vi "Bertta_v06.vi"() -> ()   [LabVIEW 2015]
uses:
  BERTTA.dll
panel:
  out "Mettler 3":dbl(graph)
  out "Mettler 2":dbl(graph)
  in  "PAUSE":bool
  in  "?":bool
  in  "Tab Control":T1(tab)
  in  "Description":string
  in  "Project name":string
  in  "User (initials)":string
  out "Mettler 1":dbl(graph)
  out "?":dbl(graph)
  in  "Balances":bool[](array[boolean])
  out "Waveform Chart 3":dynamicdata(graph)
  out "Table":string[][](table)
  in  "Headers":string[](array[string])
  in  "?":bool
  in  "Seq":dbl[][](array[numeric])=[[20.0, 60.0, 40.0], [60.0, 40.0, 20.0], [100.0, 100.0, 100.0]]
  out "Elapsed":i32
  out "Step":i32
  out "Sp":dbl
  out "T":dbl
  out "Tinit":dbl
  out "Tset":dbl
  out "Time constant":dbl
  out "Sp - Tset":i32
  out "Change":i32
  out "Waveform Chart":dynamicdata(graph)
  in  "Tbypass":dbl=33.0
  in  "Tfail":dbl=22.0
  in  "err":i32
  out "Waveform Chart 2":dynamicdata(graph)
  out "Rate (g/s)":dbl
  out "Time (s)":dbl
  out "Target (g)":dbl
  in  "Seq 2":dbl[][](array[numeric])=[[20.0, 60.0, 40.0], [60.0, 40.0, 20.0], [100.0, 100.0, 100.0]]
  out "Weight (1)":dbl
  out "target reached":i32
  out "x/y":dbl
  out "bal_previous":i32
  out "Step":i32
  in  "?":bool
  out "Step":i32
  out "bal_previous":i32
  out "x/y":dbl
  out "target reached":i32
  out "Waveform Chart 5":dynamicdata(graph)
  out "Weight (2)":dbl
  out "Rate (g/s)":dbl
  out "Time (s)":dbl
  out "Target (g)":dbl
  in  "Seq 3":dbl[][](array[numeric])=[[20.0, 60.0, 40.0], [60.0, 40.0, 20.0], [100.0, 100.0, 100.0]]
  in  "Boolean":bool
  out "Step":i32
  out "bal_previous":i32
  out "x/y":dbl
  out "target reached":i32
  out "Waveform Chart 6":dynamicdata(graph)
  out "Weight (3)":dbl
  out "Rate (g/s)":dbl
  out "Time (s)":dbl
  out "Target (g)":dbl
  in  "Seq 4":dbl[][](array[numeric])=[[20.0, 60.0, 40.0], [60.0, 40.0, 20.0], [100.0, 100.0, 100.0]]
  out "RPM":dbl
  out "Waveform Chart 4":dynamicdata(graph)
  in  "Set RPM":dbl(slide) scale=0.0..500.0
  out "Torque":dbl
  in  "?":T2(tab)
  in  "Device port":dbl=1.0
  out "Debug msg":dbl
  in  "Device port":dbl=20.0
  in  "Device port":i32=2
  in  "Device port 2":i32=6
  in  "Device port 3":i32=6
  in  "Device port 4":i32=1
  # "1"
  # "2"
  # "3"
  # "4"
  # "Step 1"
  # "Step 2"
  # "Step 3"
  # "Step 4"
  # "Step 1"
  # "Step 2"
  # "Step 3"
  # "Step 4"
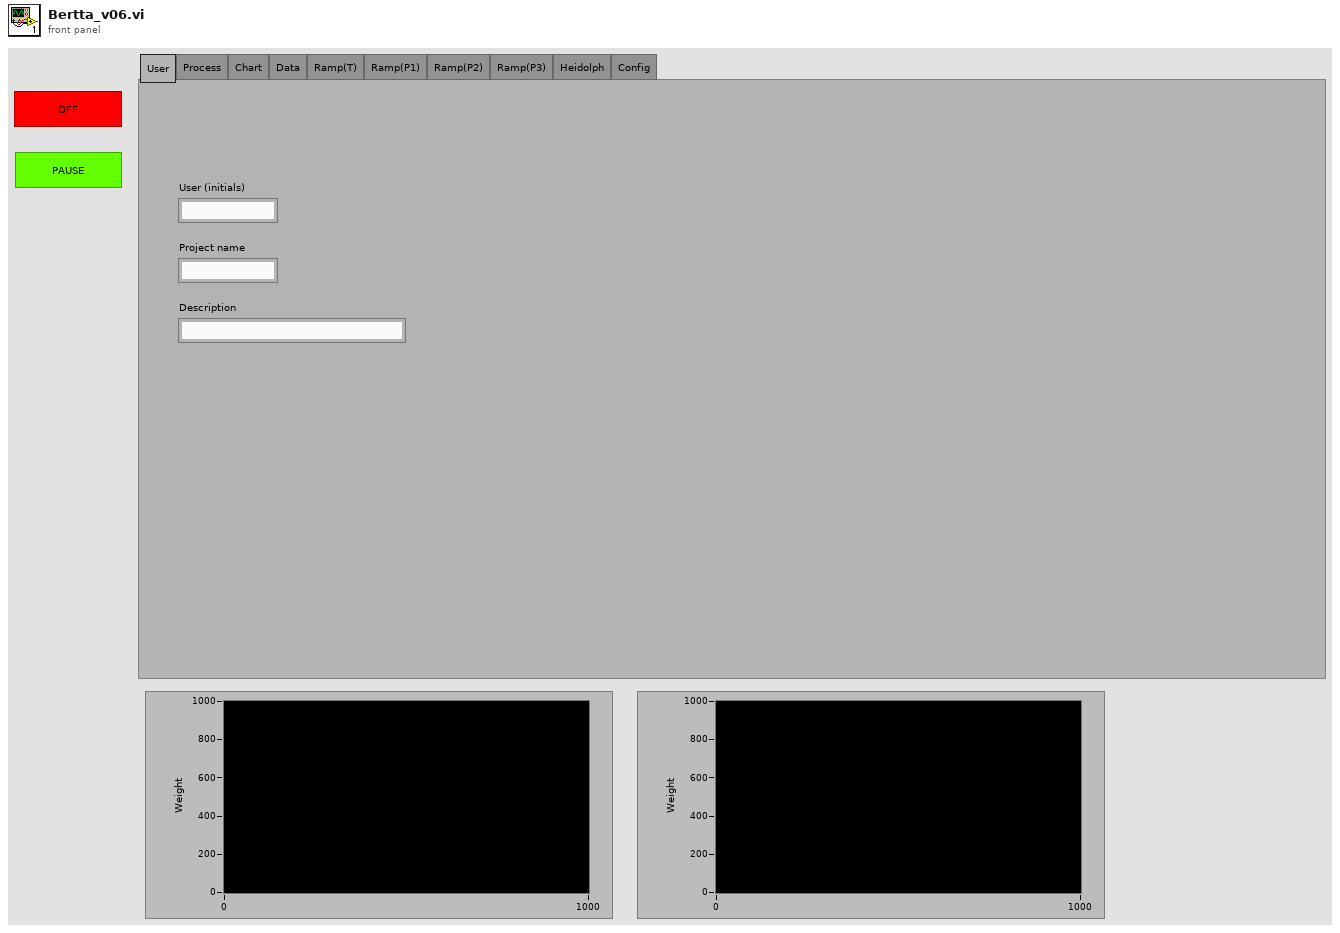
[diagram p1: front panel]
types:
  T1 = enum32{"User", "Process", "Chart", "Data", "Ramp(T)", "Ramp(P1)", "Ramp(P2)", "Ramp(P3)", "Heidolph", "Config"}
  T2 = enum32{"DB / File", "Lauda", "Heidolph", "Mettler 1", "Mettler 2", "Mettler 3", "Ismatec 1"}
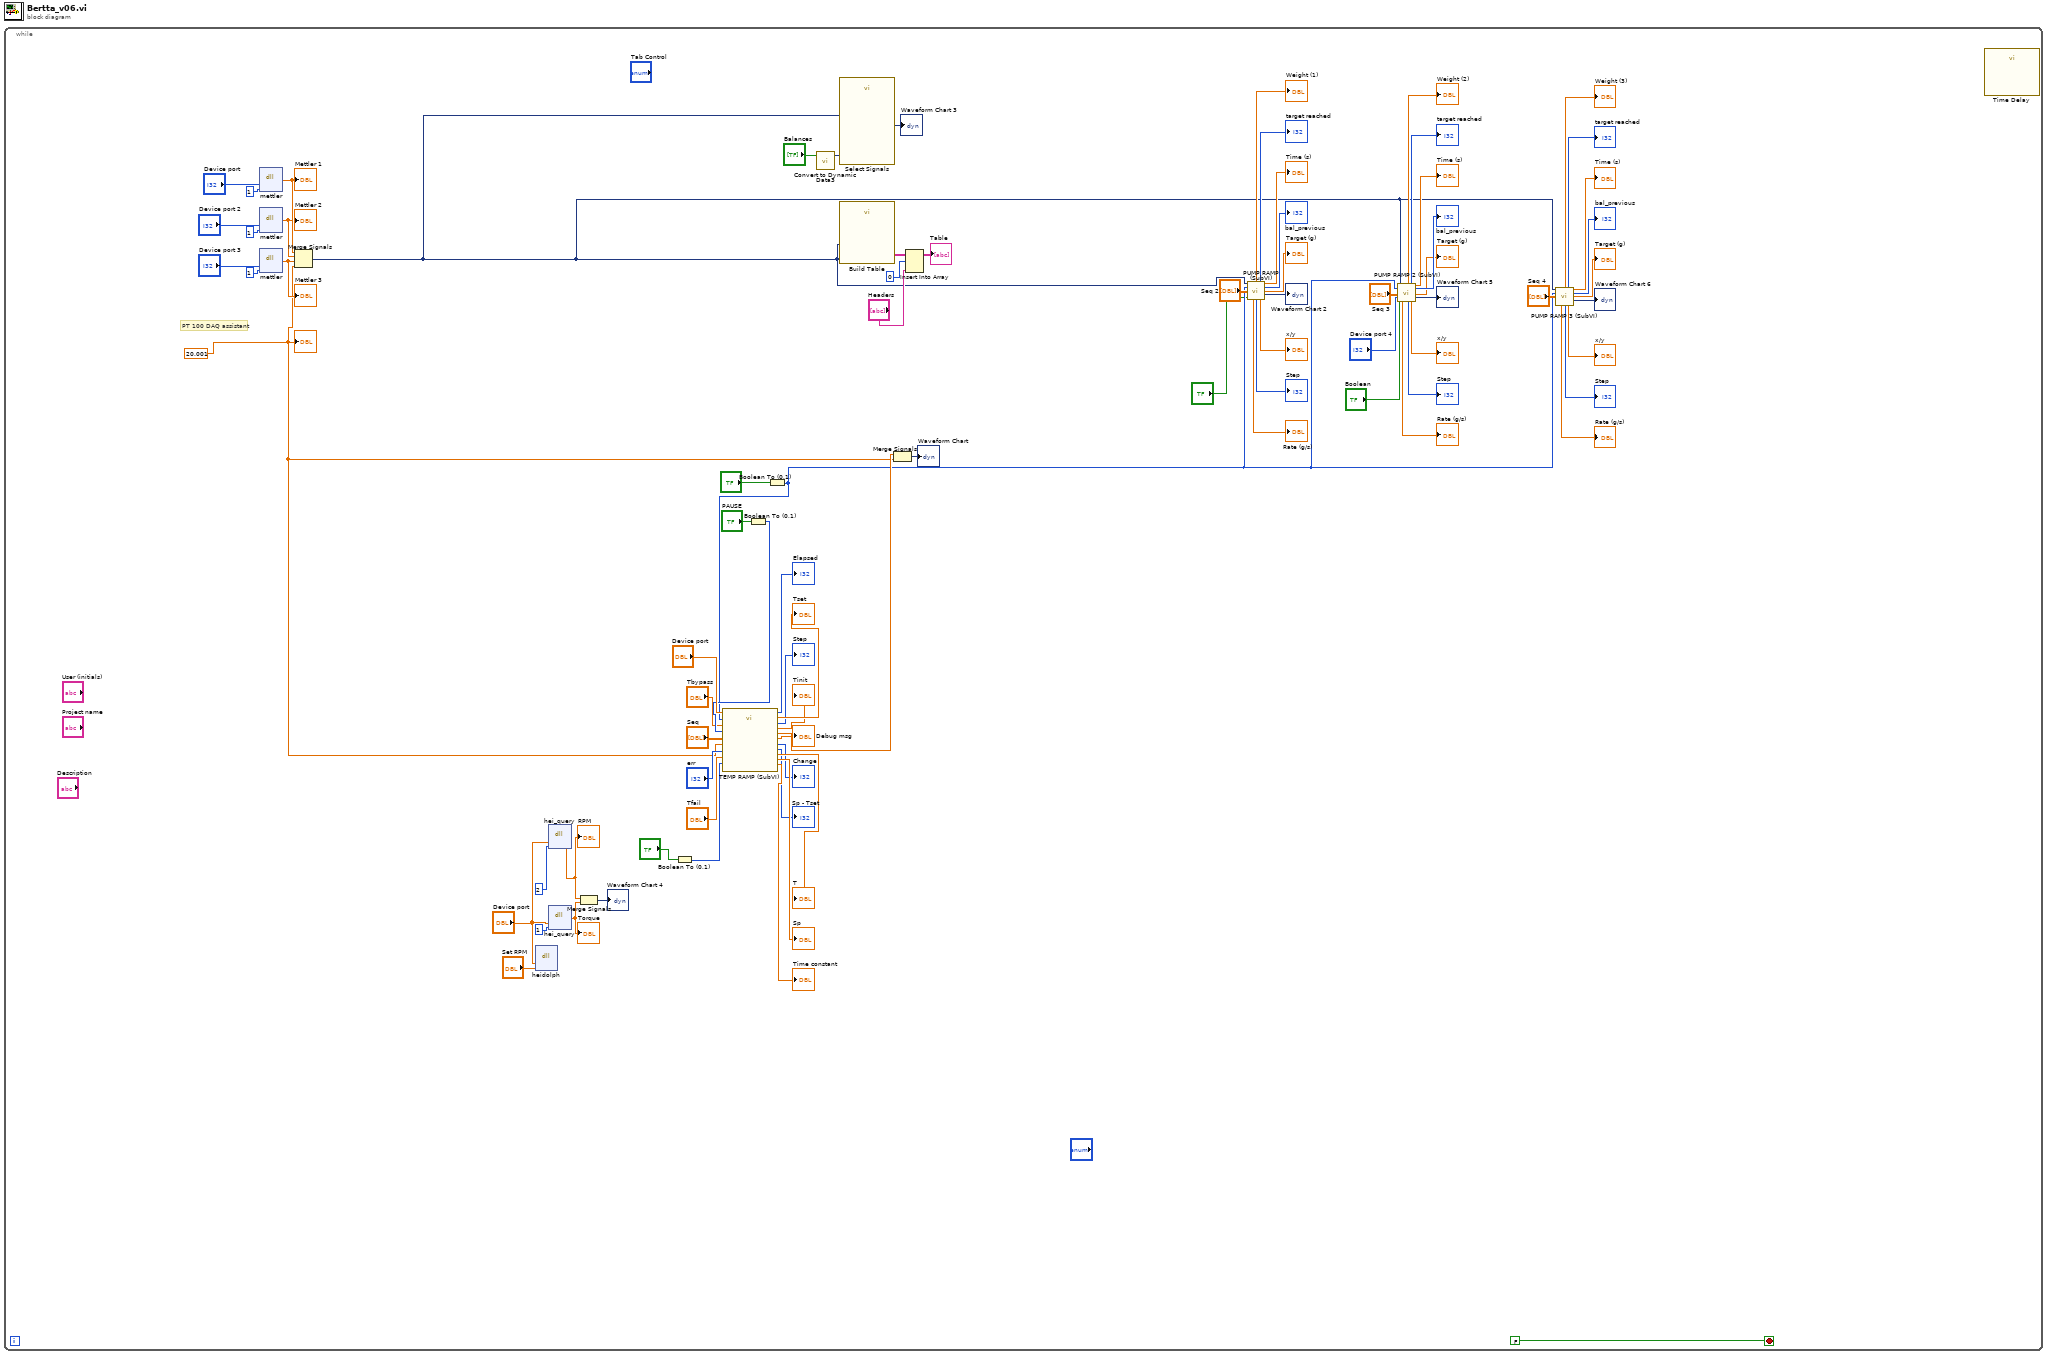
[diagram p0: block diagram]
diagram:
  n1 = while {
    stop <- FALSE stop-if-true
    w4 = 20.001
    # "PT 100 DAQ assistant"
    n2 = dll-call lib="C:/Users/xlaraser/Documents/Visual Studio 2017/Projects/Bertta/BERTTA/Debug/BERTTA.dll" fn="mettler"("port"="Device port", "msg"=1) -> ("return type"=w26:dbl)  [unwired: 5 in, 2 out]
    "Mettler 1" <- w26
    n3 = dll-call lib="C:/Users/xlaraser/Documents/Visual Studio 2017/Projects/Bertta/BERTTA/Debug/BERTTA.dll" fn="mettler"("port"="Device port 2", "msg"=1) -> ("return type"=w25:dbl)  [unwired: 5 in, 2 out]
    "Mettler 2" <- w25
    n4 = dll-call lib="C:/Users/xlaraser/Documents/Visual Studio 2017/Projects/Bertta/BERTTA/Debug/BERTTA.dll" fn="mettler"("port"="Device port 3", "msg"=1) -> ("return type"=w12:dbl)  [unwired: 5 in, 2 out]
    "Mettler 3" <- w12
    n5 = Merge Signals(w26, w25, w12, w4) -> (w5:dynamicdata)
    n6 = dll-call lib="C:/Users/xlaraser/Documents/Visual Studio 2017/Projects/Bertta/BERTTA/Debug/BERTTA.dll" fn="heidolph"("port"="Device port", "speed"="Set RPM") -> ()  [unwired: 6 in, 2 out]
    n7 = dll-call lib="C:/Users/xlaraser/Documents/Visual Studio 2017/Projects/Bertta/BERTTA/Debug/BERTTA.dll" fn="hei_query"("port"="Device port", "q"=2) -> ("return type"=w62:dbl)  [unwired: 5 in, 2 out]
    "RPM" <- w62
    n8 = dll-call lib="C:/Users/xlaraser/Documents/Visual Studio 2017/Projects/Bertta/BERTTA/Debug/BERTTA.dll" fn="hei_query"("port"="Device port", "q"=1) -> ("return type"=w61:dbl)  [unwired: 5 in, 2 out]
    "Torque" <- w61
    n9 = Merge Signals(w62, w61) -> (→"Waveform Chart 4":dynamicdata)
    n10 = Boolean To (0,1)(Boolean="?") -> (0, 1=w7:i16)
    n11 = Boolean To (0,1)(Boolean="PAUSE") -> (0, 1=w39:i16)
    n12 = Boolean To (0,1)(Boolean="?") -> (0, 1=w3:i16)
    n13 = call "TEMP RAMP (SubVI).vi"("Device port"="Device port", "Numeric"=w3, "Tbyp"="Tbypass", "Numeric 2"=w39, "Seq"="Seq", "data"=w4, "bypass"=w7, "err"="err", "Tfail"="Tfail") -> ("Sp - Tset"=→"Sp - Tset":i32, "T"=→"T":dbl, "Sp"=→"Sp":dbl, "Change"=→"Change":i32, "tr"=→"Time constant":dbl, "Debug msg"=→"Debug msg":dbl, "Elapsed"=→"Elapsed":i32, "Tset"=→"Tset":dbl, "Step"=→"Step":i32, "Tinit"=→"Tinit":dbl, "return type"=w68:dbl)
    n14 = call "Convert to Dynamic Data3"("Array"="Balances") -> ("Dynamic Data Type"=w73:dynamicdata)  [unwired: 3 in]
    n15 = call "Select Signals"("Selector Input"=w73, "Signals"=w5) -> ("Signal Out"=→"Waveform Chart 3":dynamicdata)  [unwired: 8 in, 1 out]
    n16 = call "Build Table"("Signals"=w5) -> ("Table"=w76:string[][])  [unwired: 4 in, 6 out]
    n17 = Merge Signals(w68, w4) -> (→"Waveform Chart":dynamicdata)
    n18 = Insert Into Array(array=w76, index (row)=0, new element="Headers") -> (→"Table":string[][])  [unwired: 1 in]
    n19 = call "PUMP RAMP (SubVI).vi"("Dynamic Data"=w5, "Numeric"=w3, "Seq in"="Seq 2", 11:"?") -> ("Weight (S1)"=→"Weight (1)":dbl, "target reached"=→"target reached":i32, "Time (s)"=→"Time (s)":dbl, "bal_previous"=→"bal_previous":i32, "Target (g)"=→"Target (g)":dbl, "Waveform Chart 2"=→"Waveform Chart 2":dynamicdata, "Rate (g/s)"=→"Rate (g/s)":dbl, "Step 2"=→"Step":i32, "x/y"=→"x/y":dbl)  [unwired: 3 in]
    n20 = call "PUMP RAMP 2 (SubVI).vi"("Dynamic Data"=w5, "Numeric"=w3, "Seq in"="Seq 3", "Device port"="Device port 4", "Boolean"="Boolean") -> ("Rate (g/s)"=→"Rate (g/s)":dbl, "Weight (S1)"=→"Weight (2)":dbl, "Step 2"=→"Step":i32, "target reached"=→"target reached":i32, "x/y"=→"x/y":dbl, "Time (s)"=→"Time (s)":dbl, "bal_previous"=→"bal_previous":i32, "Target (g)"=→"Target (g)":dbl, "Waveform Chart 2"=→"Waveform Chart 5":dynamicdata)  [unwired: 6 in]
    n21 = call "PUMP RAMP 3 (SubVI).vi"("Dynamic Data"=w5, "Numeric"=w3, "Seq in"="Seq 4") -> ("Weight (S1)"=→"Weight (3)":dbl, "target reached"=→"target reached":i32, "Time (s)"=→"Time (s)":dbl, "bal_previous"=→"bal_previous":i32, "Target (g)"=→"Target (g)":dbl, "Waveform Chart 2"=→"Waveform Chart 6":dynamicdata, "Rate (g/s)"=→"Rate (g/s)":dbl, "Step 2"=→"Step":i32, "x/y"=→"x/y":dbl)  [unwired: 4 in]
    n22 = call "Time Delay"() -> ()  [unwired: 11 in, 1 out]
    "?" <- w4
  }
